vi "Identify.vi"(8 "error in (no error)":errorcluster, 11 "SPI 4W Pattern Creator in":refnum<class "SPI 4W Pattern Creator.lvclass">) -> (0 "error out":errorcluster, 2 "Plugin is Valid":bool, 3 "SPI 4W Pattern Creator out":refnum<class "SPI 4W Pattern Creator.lvclass">)   [LabVIEW 2018, in "SPI 4W Pattern Creator.lvlib" / "SPI 4W Pattern Creator.lvclass"]
uses:
  SPI 4W Pattern Creator.lvclass
  C:/Users/Zijun/Desktop/zijun_PXI_dev/Solutions/5g_eap/trunk/1.0/HiSi5GmmWave/Pattern_Gen_Tool/Interfaces/Protocol Interface.lvlibp/Interfaces/Protocol Interface/Protocol Interface.lvclass
  Interfaces/Protocol Interface.lvlibp/Ctls/Protocol Type.ctl
  Interfaces/Protocol Interface.lvlibp/Interfaces/Protocol Interface/Read Protocol Type.vi
  Interfaces/Protocol Interface.lvlibp
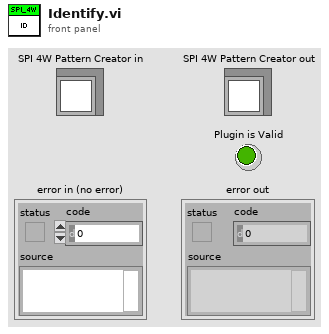
[diagram p1: front panel]
types:
  T1 = typedef "Protocol Interface.lvlibp/Protocol Type.ctl" = enum16{"BML_LS", "BML_HS", "SPI_3W", "SPI_4W"}
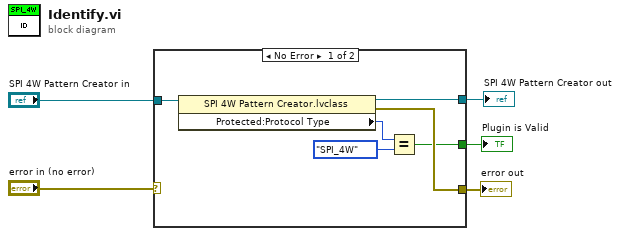
[diagram p0: block diagram]
diagram:
  n1 = case shown="No Error" "error in (no error)" {
    selector: "error in (no error)" -> [_ w12]
    tunnel: "SPI 4W Pattern Creator in" -> [w11 w13]
    tunnel: [w10 w13] -> w3
    tunnel: [w9 w12] -> w2
    tunnel: [w6 _] -> w1
    frame No Error {
      n2 = property class="SPI 4W Pattern Creator.lvclass"(reference=w11) -> (reference out=w10:refnum<class "SPI 4W Pattern Creator.lvclass">, error out=w9:errorcluster, "Protected:Protocol Type"=w8:T1)  [unwired: 1 in]
      n3 = Equal?(x=w8, y=Protocol_Type."SPI_4W") -> (x = y?=w6:bool)
    }
    frame Error {
    }
  }
  "error out" <- w2
  "SPI 4W Pattern Creator out" <- w3
  "Plugin is Valid" <- w1
